vi "dI-dV(V)_w_2w_MFLI_MF-MD_K3636B_measureR_PK_V4.0_withaveraging.vi"() -> ()   [LabVIEW 2016]
uses:
  Labview Drivers/MFLI/LabOneLabVIEW-21.02.15439/Zurich Instruments LabOne/Public/Data/ziTypeDemodSampleSingle.ctl
  Application/Labview Drivers/Keithley 2600 Series/Public/Configure/Source/Configure Source (Limit).vi
  Application/Labview Drivers/Keithley 2600 Series/Public/Configure/Source/Configure Source (Range).vi
  Labview Drivers/MFLI/LabOneLabVIEW-21.02.15439/Zurich Instruments LabOne/Public/Configure/ziGetValueDemodSampleEx.vi
  Labview Drivers/MFLI/LabOneLabVIEW-21.02.15439/Zurich Instruments LabOne/Zurich Instruments LabOne.lvlib
  Application/Labview Drivers/Keithley 2600 Series/Keithley 2600 Series.lvlib
panel:
  in  "Resistance used (ohm)":dbl=10000000.0 format="%#_13e"
  out "Direct Current (A)":dbl format="%#_13g"
  in  "Source meter K2636B (Channel A)":refnum<visa-resource-name>="GPIB0::26::INSTR"
  in  "Set Compliance current (A)":dbl=0.0001 min=0.0 step=0.1 format="%_3f"
  out "I2w vs IDC":cluster{dbl, "Field Reading":dbl}[](graph)=[{2.1337108522522826e-07, "Field Reading"=1.0007121497539348e-06}, {2.0018204953851064e-08, "Field Reading"=1.0969598663661376e-07}, {3.474074033482476e-08, "Field Reading"=1.9016075130631681e-07}, {5.6400419155691035e-08, "Field Reading"=2.706780203266455e-07}, {7.134741663483111e-08, "Field Reading"=3.625194153695155e-07}, {8.711957733763268e-08, "Field Reading"=4.6186456260881066e-07}, {1.039613386460647e-07, "Field Reading"=5.541771498802743e-07}, {1.290159481540569e-07, "Field Reading"=6.517488283090827e-07}, {1.442006622421336e-07, "Field Reading"=7.441421685111633e-07}, {1.6579779771841864e-07, "Field Reading"=8.4200282004452e-07}, {1.7667431320194624e-07, "Field Reading"=9.371894272094692e-07}, {2.0346799660082097e-07, "Field Reading"=1.0346819690568719e-06}, {2.1275449478314156e-07, "Field Reading"=1.1273455634288892e-06}, {2.2792303722372882e-07, "Field Reading"=1.2246113813938451e-06}, {2.506226161778463e-07, "Field Reading"=1.3169699353558023e-06}, {2.6686786096204173e-07, "Field Reading"=1.4106741902497636e-06}, {2.979630377408132e-07, "Field Reading"=1.5068897992871093e-06}, {3.1162936250255217e-07, "Field Reading"=1.6013785409354697e-06}, {3.2854904168138843e-07, "Field Reading"=1.7007967107121696e-06}, {3.4501678279448686e-07, "Field Reading"=1.7932741209540488e-06}, {3.5732655253185603e-07, "Field Reading"=1.891133061059139e-06}, {3.7678513716337806e-07, "Field Reading"=1.9837632139333797e-06}, {3.8857693765173823e-07, "Field Reading"=2.078638757139878e-06}, {4.070455630330932e-07, "Field Reading"=2.1777621608691614e-06}, {4.3651006057087547e-07, "Field Reading"=2.270487653250022e-06}, {4.535609885287045e-07, "Field Reading"=2.364817703267964e-06}, {4.800092323465329e-07, "Field Reading"=2.4630513126122318e-06}, {4.872172260420143e-07, "Field Reading"=2.560612214294704e-06}, {5.029105394973937e-07, "Field Reading"=2.653407522930296e-06}, {5.207137968885614e-07, "Field Reading"=2.7508846993110185e-06}, {5.449974912672081e-07, "Field Reading"=2.8437164663468094e-06}, {5.549097834910874e-07, "Field Reading"=2.941117576580943e-06}, {5.789147944756835e-07, "Field Reading"=3.0334756142859178e-06}, {5.940331669154695e-07, "Field Reading"=3.130923358288321e-06}, {6.192662248173834e-07, "Field Reading"=3.223457045619671e-06}, {6.338859460756282e-07, "Field Reading"=3.3210140787077685e-06}, {6.617730672082958e-07, "Field Reading"=3.4134337904467758e-06}, {6.708744764433933e-07, "Field Reading"=3.511218639909905e-06}, {6.876034184888421e-07, "Field Reading"=3.6064791588715936e-06}, {7.081705825683568e-07, "Field Reading"=3.704194984998823e-06}, {7.341349902267621e-07, "Field Reading"=3.796795088130521e-06}, {7.500412173627324e-07, "Field Reading"=3.894221622472711e-06}, {7.635282212201655e-07, "Field Reading"=3.986359362120525e-06}, {7.839559208505005e-07, "Field Reading"=4.084105589459172e-06}, {7.991337007295971e-07, "Field Reading"=4.176440151889332e-06}, {8.175550663233945e-07, "Field Reading"=4.274041338897146e-06}, {8.360511976155764e-07, "Field Reading"=4.366718612721536e-06}, {8.595654269642977e-07, "Field Reading"=4.46481586459238e-06}, {8.846044621269243e-07, "Field Reading"=4.559710869350914e-06}, {8.902214589762566e-07, "Field Reading"=4.6535858762473605e-06}, {9.13930972707384e-07, "Field Reading"=4.751211544539011e-06}, {9.218629476317926e-07, "Field Reading"=4.843674806906942e-06}, {9.389346568153207e-07, "Field Reading"=4.94148963023105e-06}, {9.661788530141893e-07, "Field Reading"=5.0340339305698605e-06}, {9.734275114489362e-07, "Field Reading"=5.134274890899915e-06}, {9.91273930192609e-07, "Field Reading"=5.227194198108034e-06}, {1.0062090937222443e-06, "Field Reading"=5.324543514118811e-06}, {1.0324830232331714e-06, "Field Reading"=5.417068558459935e-06}, {1.0500453704719826e-06, "Field Reading"=5.514414049876445e-06}, {1.0818020141498576e-06, "Field Reading"=5.606738838727315e-06}, {1.0919981214621985e-06, "Field Reading"=5.943499955969014e-06}, {1.1041062115858416e-06, "Field Reading"=5.802825671371831e-06}, {1.12928896400331e-06, "Field Reading"=5.8897635364887065e-06}, {1.1492595887607054e-06, "Field Reading"=5.986959246668246e-06}, {1.1525838773614565e-06, "Field Reading"=6.079112281920131e-06}, {1.1732006667255544e-06, "Field Reading"=6.176765549637453e-06}, {1.193444625294635e-06, "Field Reading"=6.2693583656248445e-06}, {1.2101538188023656e-06, "Field Reading"=6.369277338631168e-06}, {1.2318147585414787e-06, "Field Reading"=6.462177680852612e-06}, {1.2413491771177379e-06, "Field Reading"=6.554239754143973e-06}, {1.2731631837142253e-06, "Field Reading"=6.653541226069562e-06}, {1.2825564782833625e-06, "Field Reading"=6.7454110623267924e-06}, {1.2992348301055137e-06, "Field Reading"=6.843115368447837e-06}, {1.316693256967963e-06, "Field Reading"=6.935702965257668e-06}, {1.343852132299077e-06, "Field Reading"=7.033596304342718e-06}, {0.0003223256295561193, "Field Reading"=7.130369502789653e-06}, {0.0010682796466779994, "Field Reading"=7.237712618778445e-06}, {0.0011012721847992696, "Field Reading"=7.315133567183911e-06}, {0.0011336841810168491, "Field Reading"=7.4123545054478695e-06}, {0.0011614058556892847, "Field Reading"=7.504304430827025e-06}, {0.001182885890671154, "Field Reading"=7.602366955750201e-06}, {0.001200897535521615, "Field Reading"=7.69976061587441e-06}, {0.00121594401470624, "Field Reading"=7.792677109208386e-06}, {0.0012308027651267619, "Field Reading"=7.886128685028496e-06}, {0.0012456418637471253, "Field Reading"=7.983615236672288e-06}, {0.001257564969772003, "Field Reading"=8.075760842161778e-06}, {0.0012690336996615858, "Field Reading"=8.170723157183957e-06}, {0.0012814644345765262, "Field Reading"=8.268995175290895e-06}, {0.0012910253378675095, "Field Reading"=8.363131378141633e-06}, {0.001301444806581894, "Field Reading"=8.45644533427298e-06}, {0.0013106148752890106, "Field Reading"=8.551458283635111e-06}, {0.0013201336522581891, "Field Reading"=8.65161959339898e-06}, {0.0013282012490195363, "Field Reading"=8.74416723601607e-06}, {0.0013370451945670784, "Field Reading"=8.841765835802203e-06}, {0.001345475691336453, "Field Reading"=8.933978266213217e-06}, {0.0013541642420234728, "Field Reading"=9.031643266856203e-06}, {0.0013602243952778926, "Field Reading"=9.123705087732138e-06}, {0.0013678078924535615, "Field Reading"=9.221510724442928e-06}, {0.0013749931650039048, "Field Reading"=9.319154251910434e-06}, {0.0013817418853904447, "Field Reading"=9.409423170522308e-06}, {0.0013877620940512577, "Field Reading"=9.50720467327743e-06}, {0.0013893900209027232, "Field Reading"=9.522740574798281e-06}, {0.0013841293323999348, "Field Reading"=9.444358568387913e-06}, {0.0013770955503089543, "Field Reading"=9.34786117205707e-06}, {0.0013707463881856257, "Field Reading"=9.255459479065146e-06}, {0.0013638010752030354, "Field Reading"=9.157506360964617e-06}, {0.001356127430849226, "Field Reading"=9.065389480276688e-06}, {0.0013481807501391138, "Field Reading"=8.967105386552946e-06}, {0.0013407950243109453, "Field Reading"=8.872574329619889e-06}, {0.0013327879049762552, "Field Reading"=8.780745564878272e-06}, {0.0013239176518001648, "Field Reading"=8.686977265427215e-06}, {0.0013146578852826479, "Field Reading"=8.586299385882446e-06}, {0.0013048672888862206, "Field Reading"=8.493635331032656e-06}, {0.0012950842712132512, "Field Reading"=8.395823484571033e-06}, {0.0012855051336405129, "Field Reading"=8.303455420153361e-06}, {0.001274818349601112, "Field Reading"=8.209679742685101e-06}, {0.0012618971608759537, "Field Reading"=8.109946125115199e-06}, {0.0012494525821266837, "Field Reading"=8.017364894823338e-06}, {0.001235685913286103, "Field Reading"=7.919657723881713e-06}, {0.0012216877307261714, "Field Reading"=7.824897358413329e-06}, {0.0012037516065472435, "Field Reading"=7.727435253164315e-06}, {0.0011875344677767074, "Field Reading"=7.634970945479442e-06}, {0.0011690885694813937, "Field Reading"=7.537773175917453e-06}, {0.001143867923079635, "Field Reading"=7.445625913634191e-06}, {0.0011139726709101221, "Field Reading"=7.348337041113834e-06}, {0.0010813147907609588, "Field Reading"=7.255852572757193e-06}, {0.0008158901453383064, "Field Reading"=7.15654215348316e-06}, {0.00014586885402730632, "Field Reading"=7.065078532967033e-06}, {6.672313176192101e-06, "Field Reading"=6.97131792702715e-06}, {1.311378694927265e-06, "Field Reading"=6.8592321760864306e-06}, {1.318127585000335e-06, "Field Reading"=6.78165201436255e-06}, {1.2916070805813707e-06, "Field Reading"=6.684382236814962e-06}, {1.2637872492482735e-06, "Field Reading"=6.591615618281428e-06}, {1.2510857193087697e-06, "Field Reading"=6.49373019741343e-06}, {1.2409566576000475e-06, "Field Reading"=6.399307801408899e-06}, {1.215389141425889e-06, "Field Reading"=6.305912312991265e-06}, {1.1948309642776338e-06, "Field Reading"=6.211147873874382e-06}, {1.1729714746286896e-06, "Field Reading"=6.112674813622632e-06}, {1.1526746179431637e-06, "Field Reading"=6.015256707500007e-06}]
  in  "Number averaging":i32=50
  out "I2w_phase (deg)":dbl=40.57455732074348 format="%#_13g"
  out "Demod Sample Out 4":T1={"Timestamps (ticks)"=217071887690750, "X (Vrms)"=8.75456933556226e-07, "Y (Vrms)"=7.498226005787958e-07, "Osc Phase (deg)"=5.4774618983426535, "Freq (Hz)"=7.919000069023241, "DIO"=0, "AuxIn0 (V)"=-0.001673382503213361, "AuxIn1 (V)"=-0.0006673162570223212, "Trigger"=512}
  out "I2w (A)":dbl=1.1526746179431637e-06
  out "V2w_phase (deg)":dbl=40.57455732074348 format="%#_13g"
  out "Demod Sample Out 3":T1={"Timestamps (ticks)"=217071887690750, "X (Vrms)"=8.75456933556226e-07, "Y (Vrms)"=7.498226005787958e-07, "Osc Phase (deg)"=5.4774618983426535, "Freq (Hz)"=7.919000069023241, "DIO"=0, "AuxIn0 (V)"=-0.001673382503213361, "AuxIn1 (V)"=-0.0006673162570223212, "Trigger"=512}
  out "V2w (V)":dbl=1.1526746179431637e-06
  out "Iw_phase (deg)":dbl=-16.59997463839791 format="%#_13g"
  out "Vw_phase (deg)":dbl=40.57455732074348 format="%#_13g"
  out "Set Voltage(V)":dbl=4.384062043356605 format="%#_13g"
  out "Time(s)":dbl=185.322 format="%#_13g"
  out "Demod Sample Out 2":T1={"Timestamps (ticks)"=217071890701310, "X (Vrms)"=5.764492493379272e-06, "Y (Vrms)"=-1.7187028687058897e-06, "Osc Phase (deg)"=1.9746167692057917, "Freq (Hz)"=7.919000069023241, "DIO"=0, "AuxIn0 (V)"=-0.0006693530012853444, "AuxIn1 (V)"=0.0, "Trigger"=256}
  out "Demod Sample Out":T1={"Timestamps (ticks)"=217071887690750, "X (Vrms)"=8.75456933556226e-07, "Y (Vrms)"=7.498226005787958e-07, "Osc Phase (deg)"=5.4774618983426535, "Freq (Hz)"=7.919000069023241, "DIO"=0, "AuxIn0 (V)"=-0.001673382503213361, "AuxIn1 (V)"=-0.0006673162570223212, "Trigger"=512}
  in  "MFLI Current source/Voltage reader":string="DEV3647"
  out "Iw (A)":dbl=6.015256707500007e-06
  out "Vw (V)":dbl=1.1526746179431637e-06
  in  "Folder":path=path "D:/Pranava/Data/NiTe2/16-01-2022"
  in  "wait (ms) [Should be > TC]":u32=4000
  out "Vw vs IDC":cluster{dbl, "Field Reading":dbl}[](graph)=[{2.1337108522522826e-07, "Field Reading"=1.0007121497539348e-06}, {2.0018204953851064e-08, "Field Reading"=1.0969598663661376e-07}, {3.474074033482476e-08, "Field Reading"=1.9016075130631681e-07}, {5.6400419155691035e-08, "Field Reading"=2.706780203266455e-07}, {7.134741663483111e-08, "Field Reading"=3.625194153695155e-07}, {8.711957733763268e-08, "Field Reading"=4.6186456260881066e-07}, {1.039613386460647e-07, "Field Reading"=5.541771498802743e-07}, {1.290159481540569e-07, "Field Reading"=6.517488283090827e-07}, {1.442006622421336e-07, "Field Reading"=7.441421685111633e-07}, {1.6579779771841864e-07, "Field Reading"=8.4200282004452e-07}, {1.7667431320194624e-07, "Field Reading"=9.371894272094692e-07}, {2.0346799660082097e-07, "Field Reading"=1.0346819690568719e-06}, {2.1275449478314156e-07, "Field Reading"=1.1273455634288892e-06}, {2.2792303722372882e-07, "Field Reading"=1.2246113813938451e-06}, {2.506226161778463e-07, "Field Reading"=1.3169699353558023e-06}, {2.6686786096204173e-07, "Field Reading"=1.4106741902497636e-06}, {2.979630377408132e-07, "Field Reading"=1.5068897992871093e-06}, {3.1162936250255217e-07, "Field Reading"=1.6013785409354697e-06}, {3.2854904168138843e-07, "Field Reading"=1.7007967107121696e-06}, {3.4501678279448686e-07, "Field Reading"=1.7932741209540488e-06}, {3.5732655253185603e-07, "Field Reading"=1.891133061059139e-06}, {3.7678513716337806e-07, "Field Reading"=1.9837632139333797e-06}, {3.8857693765173823e-07, "Field Reading"=2.078638757139878e-06}, {4.070455630330932e-07, "Field Reading"=2.1777621608691614e-06}, {4.3651006057087547e-07, "Field Reading"=2.270487653250022e-06}, {4.535609885287045e-07, "Field Reading"=2.364817703267964e-06}, {4.800092323465329e-07, "Field Reading"=2.4630513126122318e-06}, {4.872172260420143e-07, "Field Reading"=2.560612214294704e-06}, {5.029105394973937e-07, "Field Reading"=2.653407522930296e-06}, {5.207137968885614e-07, "Field Reading"=2.7508846993110185e-06}, {5.449974912672081e-07, "Field Reading"=2.8437164663468094e-06}, {5.549097834910874e-07, "Field Reading"=2.941117576580943e-06}, {5.789147944756835e-07, "Field Reading"=3.0334756142859178e-06}, {5.940331669154695e-07, "Field Reading"=3.130923358288321e-06}, {6.192662248173834e-07, "Field Reading"=3.223457045619671e-06}, {6.338859460756282e-07, "Field Reading"=3.3210140787077685e-06}, {6.617730672082958e-07, "Field Reading"=3.4134337904467758e-06}, {6.708744764433933e-07, "Field Reading"=3.511218639909905e-06}, {6.876034184888421e-07, "Field Reading"=3.6064791588715936e-06}, {7.081705825683568e-07, "Field Reading"=3.704194984998823e-06}, {7.341349902267621e-07, "Field Reading"=3.796795088130521e-06}, {7.500412173627324e-07, "Field Reading"=3.894221622472711e-06}, {7.635282212201655e-07, "Field Reading"=3.986359362120525e-06}, {7.839559208505005e-07, "Field Reading"=4.084105589459172e-06}, {7.991337007295971e-07, "Field Reading"=4.176440151889332e-06}, {8.175550663233945e-07, "Field Reading"=4.274041338897146e-06}, {8.360511976155764e-07, "Field Reading"=4.366718612721536e-06}, {8.595654269642977e-07, "Field Reading"=4.46481586459238e-06}, {8.846044621269243e-07, "Field Reading"=4.559710869350914e-06}, {8.902214589762566e-07, "Field Reading"=4.6535858762473605e-06}, {9.13930972707384e-07, "Field Reading"=4.751211544539011e-06}, {9.218629476317926e-07, "Field Reading"=4.843674806906942e-06}, {9.389346568153207e-07, "Field Reading"=4.94148963023105e-06}, {9.661788530141893e-07, "Field Reading"=5.0340339305698605e-06}, {9.734275114489362e-07, "Field Reading"=5.134274890899915e-06}, {9.91273930192609e-07, "Field Reading"=5.227194198108034e-06}, {1.0062090937222443e-06, "Field Reading"=5.324543514118811e-06}, {1.0324830232331714e-06, "Field Reading"=5.417068558459935e-06}, {1.0500453704719826e-06, "Field Reading"=5.514414049876445e-06}, {1.0818020141498576e-06, "Field Reading"=5.606738838727315e-06}, {1.0919981214621985e-06, "Field Reading"=5.943499955969014e-06}, {1.1041062115858416e-06, "Field Reading"=5.802825671371831e-06}, {1.12928896400331e-06, "Field Reading"=5.8897635364887065e-06}, {1.1492595887607054e-06, "Field Reading"=5.986959246668246e-06}, {1.1525838773614565e-06, "Field Reading"=6.079112281920131e-06}, {1.1732006667255544e-06, "Field Reading"=6.176765549637453e-06}, {1.193444625294635e-06, "Field Reading"=6.2693583656248445e-06}, {1.2101538188023656e-06, "Field Reading"=6.369277338631168e-06}, {1.2318147585414787e-06, "Field Reading"=6.462177680852612e-06}, {1.2413491771177379e-06, "Field Reading"=6.554239754143973e-06}, {1.2731631837142253e-06, "Field Reading"=6.653541226069562e-06}, {1.2825564782833625e-06, "Field Reading"=6.7454110623267924e-06}, {1.2992348301055137e-06, "Field Reading"=6.843115368447837e-06}, {1.316693256967963e-06, "Field Reading"=6.935702965257668e-06}, {1.343852132299077e-06, "Field Reading"=7.033596304342718e-06}, {0.0003223256295561193, "Field Reading"=7.130369502789653e-06}, {0.0010682796466779994, "Field Reading"=7.237712618778445e-06}, {0.0011012721847992696, "Field Reading"=7.315133567183911e-06}, {0.0011336841810168491, "Field Reading"=7.4123545054478695e-06}, {0.0011614058556892847, "Field Reading"=7.504304430827025e-06}, {0.001182885890671154, "Field Reading"=7.602366955750201e-06}, {0.001200897535521615, "Field Reading"=7.69976061587441e-06}, {0.00121594401470624, "Field Reading"=7.792677109208386e-06}, {0.0012308027651267619, "Field Reading"=7.886128685028496e-06}, {0.0012456418637471253, "Field Reading"=7.983615236672288e-06}, {0.001257564969772003, "Field Reading"=8.075760842161778e-06}, {0.0012690336996615858, "Field Reading"=8.170723157183957e-06}, {0.0012814644345765262, "Field Reading"=8.268995175290895e-06}, {0.0012910253378675095, "Field Reading"=8.363131378141633e-06}, {0.001301444806581894, "Field Reading"=8.45644533427298e-06}, {0.0013106148752890106, "Field Reading"=8.551458283635111e-06}, {0.0013201336522581891, "Field Reading"=8.65161959339898e-06}, {0.0013282012490195363, "Field Reading"=8.74416723601607e-06}, {0.0013370451945670784, "Field Reading"=8.841765835802203e-06}, {0.001345475691336453, "Field Reading"=8.933978266213217e-06}, {0.0013541642420234728, "Field Reading"=9.031643266856203e-06}, {0.0013602243952778926, "Field Reading"=9.123705087732138e-06}, {0.0013678078924535615, "Field Reading"=9.221510724442928e-06}, {0.0013749931650039048, "Field Reading"=9.319154251910434e-06}, {0.0013817418853904447, "Field Reading"=9.409423170522308e-06}, {0.0013877620940512577, "Field Reading"=9.50720467327743e-06}, {0.0013893900209027232, "Field Reading"=9.522740574798281e-06}, {0.0013841293323999348, "Field Reading"=9.444358568387913e-06}, {0.0013770955503089543, "Field Reading"=9.34786117205707e-06}, {0.0013707463881856257, "Field Reading"=9.255459479065146e-06}, {0.0013638010752030354, "Field Reading"=9.157506360964617e-06}, {0.001356127430849226, "Field Reading"=9.065389480276688e-06}, {0.0013481807501391138, "Field Reading"=8.967105386552946e-06}, {0.0013407950243109453, "Field Reading"=8.872574329619889e-06}, {0.0013327879049762552, "Field Reading"=8.780745564878272e-06}, {0.0013239176518001648, "Field Reading"=8.686977265427215e-06}, {0.0013146578852826479, "Field Reading"=8.586299385882446e-06}, {0.0013048672888862206, "Field Reading"=8.493635331032656e-06}, {0.0012950842712132512, "Field Reading"=8.395823484571033e-06}, {0.0012855051336405129, "Field Reading"=8.303455420153361e-06}, {0.001274818349601112, "Field Reading"=8.209679742685101e-06}, {0.0012618971608759537, "Field Reading"=8.109946125115199e-06}, {0.0012494525821266837, "Field Reading"=8.017364894823338e-06}, {0.001235685913286103, "Field Reading"=7.919657723881713e-06}, {0.0012216877307261714, "Field Reading"=7.824897358413329e-06}, {0.0012037516065472435, "Field Reading"=7.727435253164315e-06}, {0.0011875344677767074, "Field Reading"=7.634970945479442e-06}, {0.0011690885694813937, "Field Reading"=7.537773175917453e-06}, {0.001143867923079635, "Field Reading"=7.445625913634191e-06}, {0.0011139726709101221, "Field Reading"=7.348337041113834e-06}, {0.0010813147907609588, "Field Reading"=7.255852572757193e-06}, {0.0008158901453383064, "Field Reading"=7.15654215348316e-06}, {0.00014586885402730632, "Field Reading"=7.065078532967033e-06}, {6.672313176192101e-06, "Field Reading"=6.97131792702715e-06}, {1.311378694927265e-06, "Field Reading"=6.8592321760864306e-06}, {1.318127585000335e-06, "Field Reading"=6.78165201436255e-06}, {1.2916070805813707e-06, "Field Reading"=6.684382236814962e-06}, {1.2637872492482735e-06, "Field Reading"=6.591615618281428e-06}, {1.2510857193087697e-06, "Field Reading"=6.49373019741343e-06}, {1.2409566576000475e-06, "Field Reading"=6.399307801408899e-06}, {1.215389141425889e-06, "Field Reading"=6.305912312991265e-06}, {1.1948309642776338e-06, "Field Reading"=6.211147873874382e-06}, {1.1729714746286896e-06, "Field Reading"=6.112674813622632e-06}, {1.1526746179431637e-06, "Field Reading"=6.015256707500007e-06}]
  out "data":dbl[](array[numeric])=[1.1526746179431637e-06, 6.015256707500007e-06, 3.1500000000000066, 184.117, 40.57455732074348, -16.59997463839791]
  in  "Step":dbl[](array[numeric])=[0.01, 0.01, 0.01] min=-3000.0 max=3000.0 format="%.1e"
  in  "To":dbl[](array[numeric])=[7.0, -7.0, 0.0] min=-3000.0 max=3000.0 format="%.1e"
  in  "From":dbl[](array[numeric])=[0.0, 7.0, -7.0] min=-3000.0 max=3000.0 format="%.1e"
  in  "file name":string="001_NiTe2_13-12-2021_DeviceB_I_31-33_V_30-35_dI_dV (DC_V)+second_harmonic_K2636B_10Mohmbuffer_7.919Hz_7mK_ZF_50ave"
  out "File path":path=path "D:/Heng/Nb3Br8_JJ/Sb.3_NBVJ01/20210115/002_NBVJ01_IV(8mK)_I16_R34_ac(13.3337Hz).dat"
  # ".dat"
  # "Set MFLI Voltage output (V)"
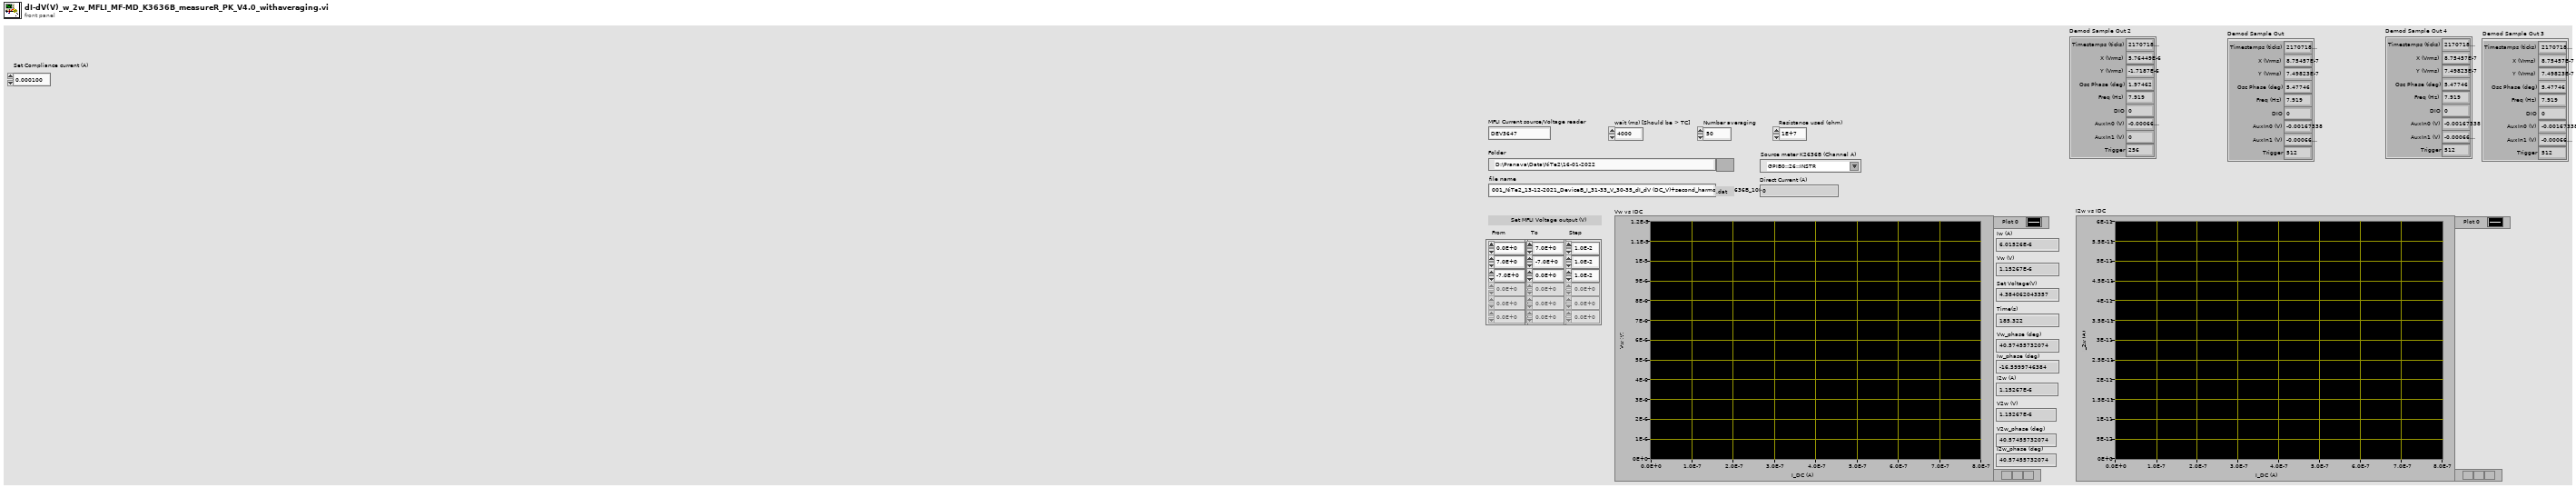
[diagram p1: front panel]
types:
  T1 = typedef "Zurich Instruments LabOne.lvlib/ziTypeDemodSampleSingle.ctl" = cluster{"Timestamps (ticks)":u64, "X (Vrms)":dbl, "Y (Vrms)":dbl, "Osc Phase (deg)":dbl, "Freq (Hz)":dbl, "DIO":u32, "AuxIn0 (V)":dbl, "AuxIn1 (V)":dbl, "Trigger":u32}
  T2 = enum16{"open", "replace", "create", "open or create", "replace or create", "replace or create with confirmation"}
  T3 = typedef "Zurich Instruments LabOne.lvlib/ziTypeHandle.ctl" = cluster{"handleValid":bool, "Conn":u64, "Path Prefix":string, "Handle":u64, "Connected":bool, "Clockbase(s)":dbl}
  T4 = cluster{"Direct Current (A)":dbl, "Average value":dbl}
  T5 = cluster{"Direct Current (A)":dbl, "Average value":dbl}[]
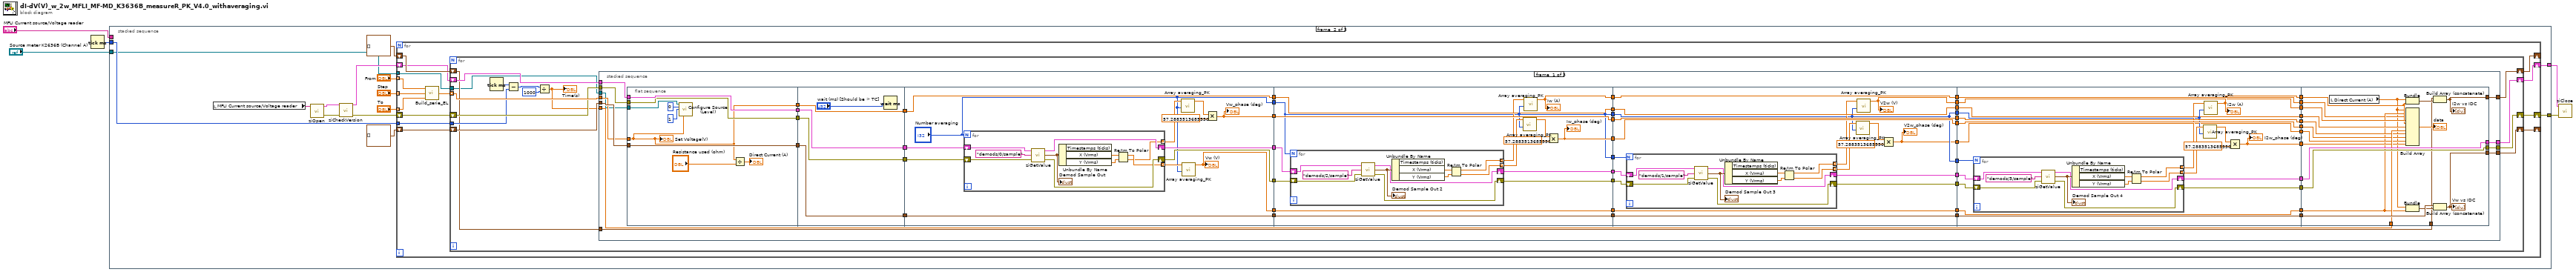
[diagram p0: block diagram]
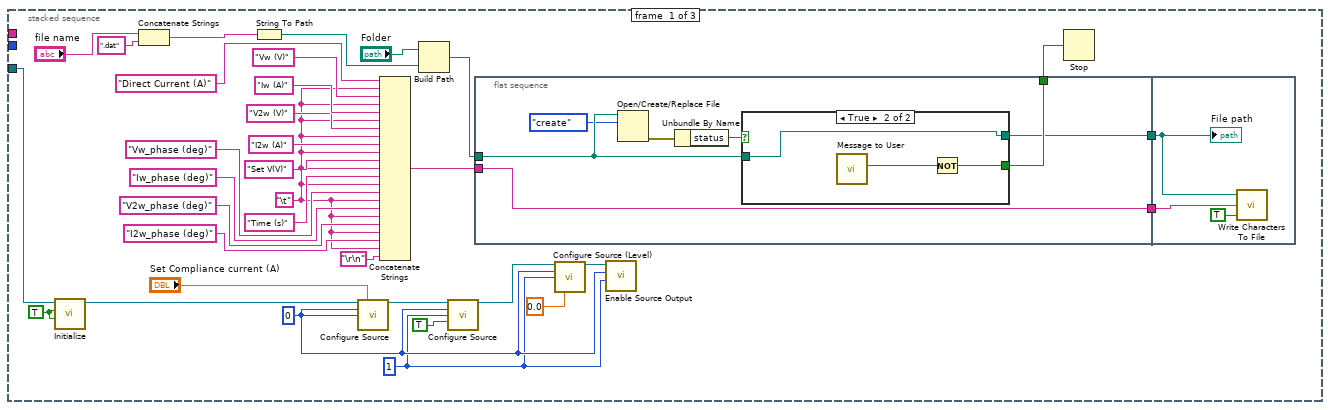
[diagram p2: hidden frame]
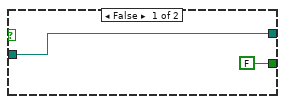
[diagram p3: hidden frame]
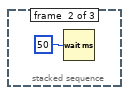
[diagram p4: hidden frame]
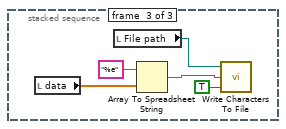
[diagram p5: hidden frame]
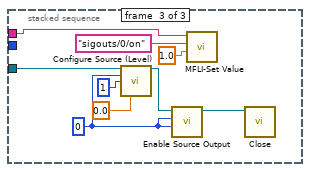
[diagram p6: hidden frame]
diagram:
  n1 = Tick Count (ms)() -> (millisecond timer value=w4:u32)
  n2 = stacked-sequence {
    tunnel: "MFLI Current source/Voltage reader" -> [_ _ w310]
    tunnel: w4 -> [_ w64 _]
    tunnel: [_ w62 _] -> w3
    tunnel: [_ w61 _] -> w2
    tunnel: "Source meter K2636B (Channel A)" -> [w9 w55 w304]
    frame #0 {
      w11 = TRUE
      w14 = 0
      w12 = 1
      w6 = "\t"
      n3 = call "Initialize.vi"("Reset (True)"=w11, "ID Query (True)"=w11, "VISA resource name"=w9) -> ("VISA resource name out"=w8:refnum<visa-resource-name>)  [unwired: 7 in, 1 out]
      n4 = Concatenate Strings("file name", ".dat" ("string")) -> (w36:string)
      n5 = String To Path(string=w36) -> (path=w29:path)
      n6 = call-poly "Configure Source.vi"("VISA resource name"=w8, "Current Limit (0.1 A)"="Set Compliance current (A)", "Source Measure Unit Channel (0: Channel A)"=w14, "Limit Type (1: Voltage)"=w14) -> ("VISA resource name out"=w18:refnum<visa-resource-name>)  [unwired: 10 in, 1 out]
      n7 = Concatenate Strings("Direct Current (A)", w6, "Vw (V)" ("string"), w6, "Iw (A)" ("string"), w6, "V2w (V)" ("string"), w6, "I2w (A)" ("string"), w6, "Set V(V)" ("string"), w6, "Time (s)", w6, "Vw_phase (deg)", w6, "Iw_phase (deg)", w6, "V2w_phase (deg)", w6, "I2w_phase (deg)", w6, "\r\n") -> (w37:string)
      n8 = Build Path(base path="Folder", name or relative path=w29) -> (appended path=w28:path)
      n9 = call-poly "Configure Source.vi"("VISA resource name"=w18, "Source Measure Unit Channel (0: Channel A)"=w14, "Range Type (1: Voltage)"=w12, "Auto Range (T: Enable)"=TRUE) -> ("VISA resource name out"=w17:refnum<visa-resource-name>)  [unwired: 10 in, 1 out]
      n10 = flat-sequence {
        tunnel: w28 -> [w43]
        tunnel: w37 -> [w46]
        tunnel: [w46] -> w39
        tunnel: [w45] -> w34
        tunnel: [w44] -> w38
        tunnel: w39 -> [w53]
        tunnel: w38 -> [w52]
        frame #0 {
          n11 = Open/Create/Replace File(file path (use dialog)=w43, operation (0:open)=T2."create") -> (error out=w42:errorcluster)  [unwired: 4 in, 2 out]
          n12 = Unbundle By Name(w42) -> ("status"=w40:bool)
          n13 = case shown="True" w40 {
            tunnel: [FALSE ("Yes") w50] -> w45
            tunnel: [w47 w49] -> w44
            tunnel: w43 -> [w47 w49]
            frame False {
            }
            frame True {
              n14 = call "Message to User"() -> ("Yes"=w51:bool)  [unwired: 10 in, 1 out]
              n15 = Not(x=w51) -> (.not. x?=w50:bool)
            }
          }
        }
        frame #1 {
          n16 = call <vilib>:"Write Characters To File.vi"("append to file? (new file:F)"=TRUE, "character string"=w53, "file path (dialog if empty)"=w52) -> ()  [unwired: 2 in, 1 out]
          "File path" <- w52
        }
      }
      n17 = call "Configure Source (Level).vi"("VISA resource name"=w17, "Source Measure Unit Channel (0: Channel A)"=w14, "Level Type (1: Voltage)"=w12, "Voltage Level (0 V)"=0.0) -> ("VISA resource name out"=w16:refnum<visa-resource-name>)  [unwired: 10 in, 1 out]
      n18 = call "Enable Source Output.vi"("Output Mode (0: Turn off)"=w12, "Source Measure Unit Channel (0: Channel A)"=w14, "VISA resource name"=w16) -> ()  [unwired: 7 in, 2 out]
      n19 = Stop(stop? (T)=w34) -> ()
    }
    frame #1 {
      n20 = local read "MFLI Current source/Voltage reader"() -> (w58:string)
      n21 = call "ziOpen.vi"("Address"=w58) -> ("Error Out"=w59:errorcluster, "HandleOut"=w60:T3)  [unwired: 3 in, 1 out]
      n22 = call "ziCheckVersion.vi"("Handle In"=w60, "Error In"=w59) -> ("Handle Out"=w57:T3, "Error Out"=w56:errorcluster)  [unwired: 11 in, 1 out]
      n23 = for {
        tunnel: "From" -> [w79] mode=indexing
        tunnel: "To" -> [w78] mode=indexing
        tunnel: "Step" -> [w77] mode=indexing
        shift-right: [w81] -> _
        shift-left: cluster{dbl, "Field Reading":dbl}[] [] -> [w82]
        tunnel: w64 -> [w76]
        shift-right: [w75] -> _
        shift-left: cluster{dbl, "Field Reading":dbl}[] [] -> [w74]
        shift-right: [w73] -> w62
        shift-left: w57 -> [w71]
        shift-right: [w72] -> w61
        shift-left: w56 -> [w70]
        tunnel: w55 -> [w69]
        n24 = call "Build_serie_EL.vi"("end value"=w78, "increment"=w77, "start value"=w79) -> ("output array"=w80:dbl[])
        n25 = for {
          tunnel: w80 -> [w97] mode=indexing
          shift-right: [w95] -> w81
          shift-left: w82 -> [w96]
          shift-right: [w92] -> w73
          shift-left: w71 -> [w94]
          shift-right: [w91] -> w72
          shift-left: w70 -> [w93]
          tunnel: w76 -> [w87]
          shift-right: [w85] -> w75
          shift-left: w74 -> [w84]
          tunnel: w69 -> [w83]
          n26 = Tick Count (ms)() -> (millisecond timer value=w88:u32)
          n27 = Subtract(x=w88, y=w87) -> (x-y=w89:u32)
          n28 = Divide(x=w89, y=1000) -> (x/y=w86:dbl)
          "Time(s)" <- w86
          n29 = stacked-sequence {
            tunnel: w97 -> [w155 _ _]
            tunnel: w96 -> [w156 _ _]
            tunnel: [w157 _ _] -> w95
            tunnel: w94 -> [w147 _ _]
            tunnel: w93 -> [w146 _ _]
            tunnel: [w140 _ _] -> w92
            tunnel: [w139 _ _] -> w91
            tunnel: w86 -> [w138 _ _]
            tunnel: [w101 _ _] -> w85
            tunnel: w84 -> [w100 _ _]
            tunnel: w83 -> [w98 _ _]
            frame #0 {
              n30 = flat-sequence {
                tunnel: [w166] -> w152
                tunnel: [w160] -> w151
                tunnel: w155 -> [w160]
                tunnel: w156 -> [w166]
                tunnel: [w163] -> w148
                tunnel: w147 -> [w163]
                tunnel: w146 -> [w162]
                tunnel: [w162] -> w99
                tunnel: w98 -> [w161]
                tunnel: w152 -> [w171]
                tunnel: [w171] -> w154
                tunnel: w151 -> [w170]
                tunnel: [w170] -> w153
                tunnel: [w168] -> w150
                tunnel: [w167] -> w149
                tunnel: w148 -> [w168]
                tunnel: w99 -> [w167]
                tunnel: [w176] -> w145
                tunnel: [w184] -> w144
                tunnel: [w183] -> w143
                tunnel: w149 -> [w182]
                tunnel: w150 -> [w181]
                tunnel: w154 -> [w184]
                tunnel: w153 -> [w183]
                tunnel: [w180] -> w142
                tunnel: [w179] -> w141
                tunnel: [w178] -> w137
                tunnel: ["Number averaging"] -> w114
                tunnel: w145 -> [w203]
                tunnel: [w203] -> w136
                tunnel: w144 -> [w209]
                tunnel: [w209] -> w135
                tunnel: w143 -> [w208]
                tunnel: [w208] -> w134
                tunnel: w142 -> [w207]
                tunnel: w141 -> [w206]
                tunnel: [w205] -> w133
                tunnel: [w204] -> w132
                tunnel: [w199] -> w131
                tunnel: [w200] -> w130
                tunnel: w137 -> [w202]
                tunnel: [w202] -> w129
                tunnel: w114 -> [w195]
                tunnel: [w195] -> w112
                tunnel: [w195] -> w111
                tunnel: w136 -> [w237]
                tunnel: [w237] -> w128
                tunnel: w135 -> [w236]
                tunnel: [w236] -> w126
                tunnel: w134 -> [w235]
                tunnel: [w235] -> w124
                tunnel: w133 -> [w230]
                tunnel: w132 -> [w229]
                tunnel: [w224] -> w122
                tunnel: w131 -> [w234]
                tunnel: [w234] -> w120
                tunnel: w130 -> [w233]
                tunnel: [w233] -> w118
                tunnel: w129 -> [w232]
                tunnel: [w232] -> w116
                tunnel: [w225] -> w113
                tunnel: w112 -> [w223]
                tunnel: w111 -> [w222]
                tunnel: [w222] -> w109
                tunnel: [w222] -> w108
                tunnel: [w221] -> w106
                tunnel: [w220] -> w103
                tunnel: w128 -> [w267]
                tunnel: [w267] -> w127
                tunnel: w126 -> [w266]
                tunnel: [w266] -> w125
                tunnel: w124 -> [w265]
                tunnel: [w265] -> w123
                tunnel: w122 -> [w259]
                tunnel: [w257] -> w121
                tunnel: w120 -> [w264]
                tunnel: [w264] -> w119
                tunnel: w118 -> [w263]
                tunnel: [w263] -> w117
                tunnel: w116 -> [w262]
                tunnel: [w262] -> w115
                tunnel: w113 -> [w260]
                tunnel: [w258] -> w110
                tunnel: w109 -> [w253]
                tunnel: w108 -> [w252]
                tunnel: [w251] -> w107
                tunnel: w106 -> [w250]
                tunnel: [w250] -> w105
                tunnel: [w249] -> w104
                tunnel: w103 -> [w248]
                tunnel: [w248] -> w102
                tunnel: w127 -> [w281]
                tunnel: [w296] -> w157
                tunnel: w125 -> [w295]
                tunnel: w123 -> [w283]
                tunnel: [w294] -> w140
                tunnel: [w293] -> w139
                tunnel: w121 -> [w293]
                tunnel: w119 -> [w280]
                tunnel: w138 -> [w291]
                tunnel: w117 -> [w290]
                tunnel: w115 -> [w289]
                tunnel: w110 -> [w294]
                tunnel: w107 -> [w282]
                tunnel: w105 -> [w288]
                tunnel: w104 -> [w287]
                tunnel: w102 -> [w286]
                tunnel: [w284] -> w101
                tunnel: w100 -> [w279]
                frame #0 {
                  n31 = call "Configure Source (Level).vi"("VISA resource name"=w161, "Source Measure Unit Channel (0: Channel A)"=0, "Level Type (1: Voltage)"=1, "Voltage Level (0 V)"=w160) -> ()  [unwired: 10 in, 2 out]
                  n32 = Divide(x=w160, y="Resistance used (ohm)") -> (x/y=→"Direct Current (A)":dbl)
                  "Set Voltage(V)" <- w160
                }
                frame #1 {
                  n33 = Wait (ms)(milliseconds to wait="wait (ms) [Should be > TC]") -> ()  [unwired: 1 out]
                }
                frame #2 {
                  n34 = for {
                    N: "Number averaging" -> [_]
                    tunnel: [w186] -> w175 mode=indexing
                    tunnel: [w185] -> w173 mode=indexing
                    shift-right: [w189] -> w179
                    shift-left: w182 -> [w192]
                    shift-right: [w190] -> w180
                    shift-left: w181 -> [w191]
                    n35 = call-poly "ziGetValue.vi"("error in"=w192, "Path"="demods/0/sample", "Handle In"=w191) -> ("error out"=w189:errorcluster, "Demod Sample Out"=w193:T1, "Handle Out"=w190:T3)
                    "Demod Sample Out" <- w193
                    n36 = Unbundle By Name(w193) -> ("X (Vrms)"=w188:dbl, "Y (Vrms)"=w187:dbl)  [unwired: 1 out]
                    n37 = Re/Im To Polar(2:w187, 3:w188) -> (0:w185:dbl, 1:w186:dbl)
                  }
                  n38 = call "Array averaging_PK.vi"("Number averaging"="Number averaging", "numeric array"=w173) -> ("Average value"=w174:dbl)  [unwired: 9 in]
                  n39 = call "Array averaging_PK.vi"("Number averaging"="Number averaging", "numeric array"=w175) -> ("Average value"=w176:dbl)  [unwired: 9 in]
                  "Vw (V)" <- w176
                  n40 = Multiply(x=w174, y=57.28835136855506) -> (x*y=w178:dbl)
                  "Vw_phase (deg)" <- w178
                }
                frame #3 {
                  n41 = for {
                    N: w195 -> [_]
                    tunnel: [w211] -> w197 mode=indexing
                    tunnel: [w210] -> w196 mode=indexing
                    shift-right: [w215] -> w205
                    shift-left: w207 -> [w217]
                    shift-right: [w214] -> w204
                    shift-left: w206 -> [w216]
                    n42 = call-poly "ziGetValue.vi"("error in"=w216, "Path"="demods/2/sample", "Handle In"=w217) -> ("error out"=w214:errorcluster, "Demod Sample Out"=w218:T1, "Handle Out"=w215:T3)
                    "Demod Sample Out 2" <- w218
                    n43 = Unbundle By Name(w218) -> ("X (Vrms)"=w212:dbl, "Y (Vrms)"=w213:dbl)  [unwired: 1 out]
                    n44 = Re/Im To Polar(2:w213, 3:w212) -> (0:w210:dbl, 1:w211:dbl)
                  }
                  n45 = call "Array averaging_PK.vi"("Number averaging"=w195, "numeric array"=w196) -> ("Average value"=w198:dbl)  [unwired: 9 in]
                  n46 = call "Array averaging_PK.vi"("Number averaging"=w195, "numeric array"=w197) -> ("Average value"=w199:dbl)  [unwired: 9 in]
                  "Iw (A)" <- w199
                  n47 = Multiply(x=w198, y=57.28835136855506) -> (x*y=w200:dbl)
                  "Iw_phase (deg)" <- w200
                }
                frame #4 {
                  n48 = for {
                    N: w223 -> [_]
                    tunnel: [w243] -> w226 mode=indexing
                    tunnel: [w242] -> w228 mode=indexing
                    shift-right: [w239] -> w225
                    shift-left: w230 -> [w241]
                    shift-right: [w238] -> w224
                    shift-left: w229 -> [w240]
                    n49 = call-poly "ziGetValue.vi"("error in"=w240, "Path"="demods/1/sample", "Handle In"=w241) -> ("error out"=w238:errorcluster, "Demod Sample Out"=w246:T1, "Handle Out"=w239:T3)
                    "Demod Sample Out 3" <- w246
                    n50 = Unbundle By Name(w246) -> ("X (Vrms)"=w245:dbl, "Y (Vrms)"=w244:dbl)  [unwired: 1 out]
                    n51 = Re/Im To Polar(2:w244, 3:w245) -> (0:w242:dbl, 1:w243:dbl)
                  }
                  n52 = call "Array averaging_PK.vi"("Number averaging"=w222, "numeric array"=w228) -> ("Average value"=w227:dbl)  [unwired: 9 in]
                  n53 = call "Array averaging_PK.vi"("Number averaging"=w222, "numeric array"=w226) -> ("Average value"=w221:dbl)  [unwired: 9 in]
                  "V2w (V)" <- w221
                  n54 = Multiply(x=w227, y=57.28835136855506) -> (x*y=w220:dbl)
                  "V2w_phase (deg)" <- w220
                }
                frame #5 {
                  n55 = for {
                    N: w253 -> [_]
                    tunnel: [w273] -> w256 mode=indexing
                    tunnel: [w272] -> w254 mode=indexing
                    shift-right: [w269] -> w258
                    shift-left: w260 -> [w271]
                    shift-right: [w268] -> w257
                    shift-left: w259 -> [w270]
                    n56 = call-poly "ziGetValue.vi"("error in"=w270, "Path"="demods/3/sample", "Handle In"=w271) -> ("error out"=w268:errorcluster, "Demod Sample Out"=w276:T1, "Handle Out"=w269:T3)
                    "Demod Sample Out 4" <- w276
                    n57 = Unbundle By Name(w276) -> ("X (Vrms)"=w275:dbl, "Y (Vrms)"=w274:dbl)  [unwired: 1 out]
                    n58 = Re/Im To Polar(2:w274, 3:w275) -> (0:w272:dbl, 1:w273:dbl)
                  }
                  n59 = call "Array averaging_PK.vi"("Number averaging"=w252, "numeric array"=w254) -> ("Average value"=w255:dbl)  [unwired: 9 in]
                  n60 = call "Array averaging_PK.vi"("Number averaging"=w252, "numeric array"=w256) -> ("Average value"=w251:dbl)  [unwired: 9 in]
                  "I2w (A)" <- w251
                  n61 = Multiply(x=w255, y=57.28835136855506) -> (x*y=w249:dbl)
                  "I2w_phase (deg)" <- w249
                }
                frame #6 {
                  n62 = local read "Direct Current (A)"() -> (w278:dbl)
                  n63 = Bundle("Direct Current (A)"=w278, "Average value"=w282) -> (w285:T4)  [unwired: 1 in]
                  n64 = Build Array(w278, w281, w280, w288, w282, w283, w291, w289, w290, w286, w287) -> (→"data":dbl[])
                  n65 = Bundle("Direct Current (A)"=w278, "Average value"=w281) -> (w292:T4)  [unwired: 1 in]
                  n66 = Build Array (concatenate)(w279, w285) -> (w284:T5)
                  "I2w vs IDC" <- w284
                  n67 = Build Array (concatenate)(w295, w292) -> (w296:T5)
                  "Vw vs IDC" <- w296
                }
              }
            }
            frame #1 {
              n68 = Wait (ms)(milliseconds to wait=u32 50) -> ()  [unwired: 1 out]
            }
            frame #2 {
              n69 = local read "data"() -> (w299:dbl[])
              n70 = local read "File path"() -> (w301:path)
              n71 = Array To Spreadsheet String(array=w299, 3:"%e" ("format string")) -> (spreadsheet string=w302:string)  [unwired: 1 in]
              n72 = call <vilib>:"Write Characters To File.vi"("append to file? (new file:F)"=TRUE, "character string"=w302, "file path (dialog if empty)"=w301) -> ()  [unwired: 2 in, 1 out]
            }
          }
        }
      }
    }
    frame #2 {
      w307 = 0
      n73 = call "Configure Source (Level).vi"("VISA resource name"=w304, "Source Measure Unit Channel (0: Channel A)"=w307, "Level Type (1: Voltage)"=1, "Voltage Level (0 V)"=0.0) -> ("VISA resource name out"=w309:refnum<visa-resource-name>)  [unwired: 10 in, 1 out]
      n74 = call "Enable Source Output.vi"("Output Mode (0: Turn off)"=w307, "Source Measure Unit Channel (0: Channel A)"=w307, "VISA resource name"=w309) -> ("VISA resource name out"=w305:refnum<visa-resource-name>)  [unwired: 7 in, 1 out]
      n75 = call "MFLI-Set Value.vi"("Value"=1.0, "Path"="sigouts/0/on", "MFLI Current source/Voltage reader"=w310) -> ()  [unwired: 9 in]
      n76 = call "Close.vi"("VISA resource name"=w305) -> ()  [unwired: 10 in, 1 out]
    }
  }
  n77 = call "ziClose.vi"("Error In"=w2, "Handle In"=w3) -> ()  [unwired: 4 out]
